vi "Clamp Range.vi"(1 "Min":dbl, 2 "Value":dbl, 3 "Bias":dbl, 4 "Max":dbl) -> (0 "Output":dbl)   [LabVIEW 2016]
panel:
  # "Keeps sign of original value, and keeps value in range with bias"
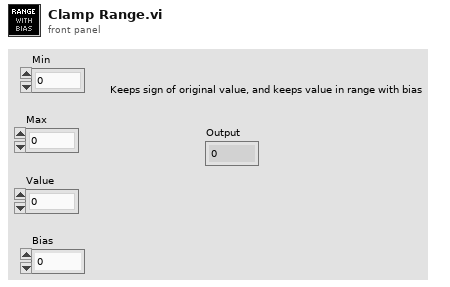
[diagram p1: front panel]
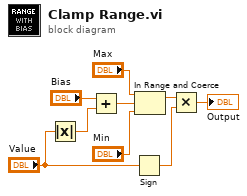
[diagram p0: block diagram]
diagram:
  n1 = Absolute Value(x="Value") -> (abs(x)=w9:dbl)
  n2 = Add(x="Bias", y=w9) -> (x+y=w5:dbl)
  n3 = Sign(1:"Value") -> (0:w2:dbl)
  n4 = In Range and Coerce(upper limit="Max", x=w5, lower limit="Min") -> (coerced(x)=w4:dbl)  [unwired: 1 out]
  n5 = Multiply(x=w4, y=w2) -> (x*y=→"Output":dbl)
